vi "Calculate Average Center.vi"(10 "Position":i32, 11 "Gantry Fiducials":dbl[](array[numeric])) -> (2 "Array":cluster{"X":sgl, "Y":sgl}[](array[cluster]), 3 "XYZTheta":dbl[](array[numeric]))   [LabVIEW 2020, in "Assembly Tray.lvclass"]
uses:
  Assembly Tray.lvclass
  <vilib>/Analysis/NI_AALBase.lvlib
  <vilib>/Analysis/baseanly.llb/Mean (DBL).vi
  <vilib>/vision/NI_Vision_Development_Module.lvlib
panel:
  in  "Line 1":T1
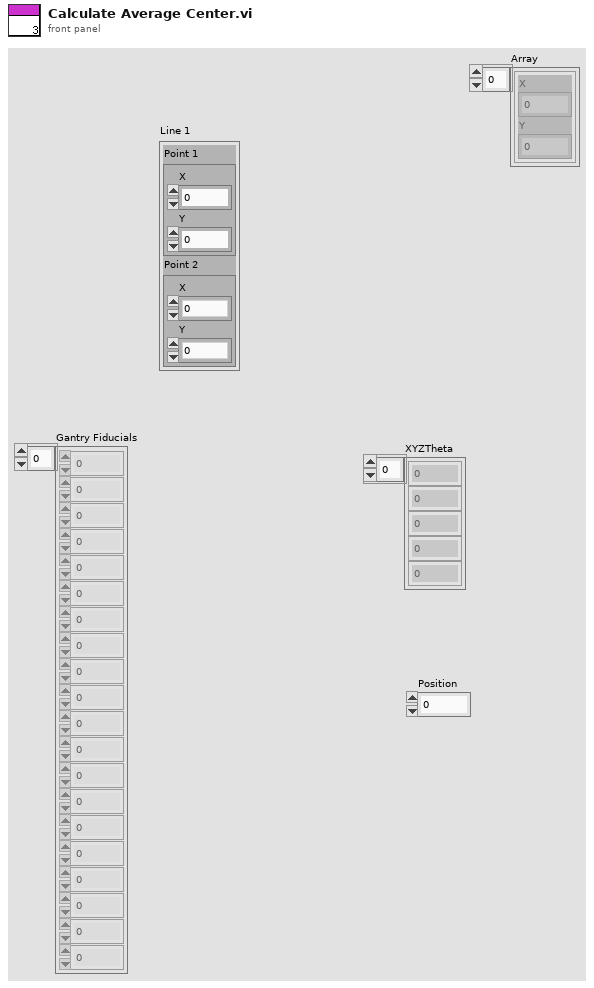
[diagram p1: front panel]
types:
  T1 = cluster{"Point 1":cluster{"X":dbl, "Y":dbl}, "Point 2":cluster{"X":dbl, "Y":dbl}}
  T2 = cluster{"Point 1":cluster{"X":dbl, "Y":dbl}, "Point 2":cluster{"X":dbl, "Y":dbl}}[]
  T3 = cluster{"Point 1":cluster{"X":dbl, "Y":dbl}, "Point 2":cluster{"X":dbl, "Y":dbl}}[][]
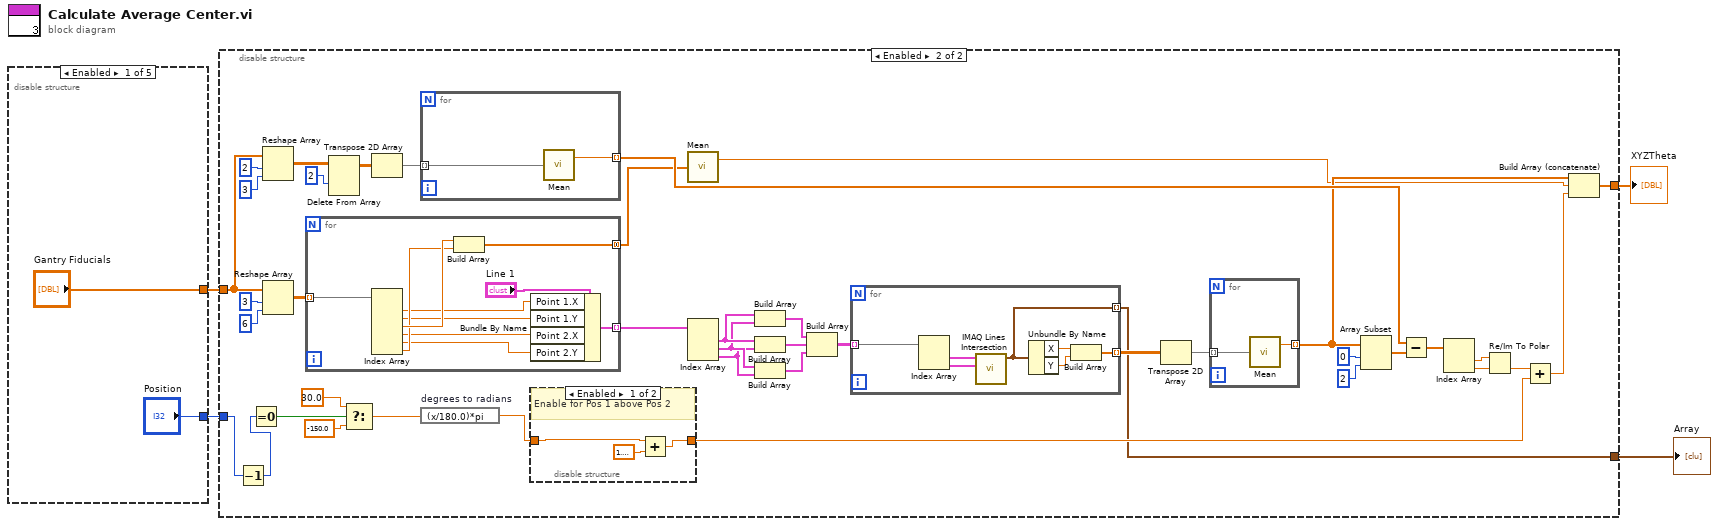
[diagram p0: block diagram]
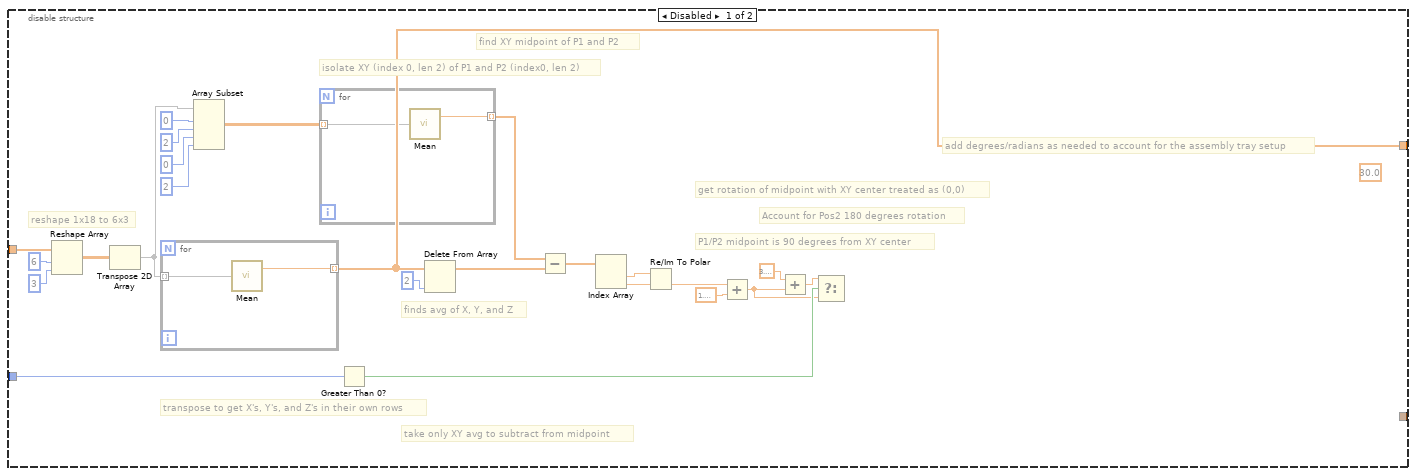
[diagram p2: hidden frame]
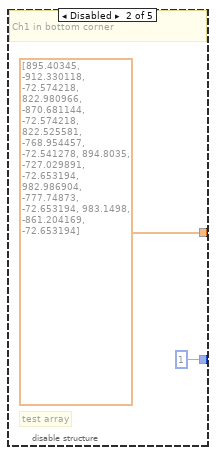
[diagram p4: hidden frame]
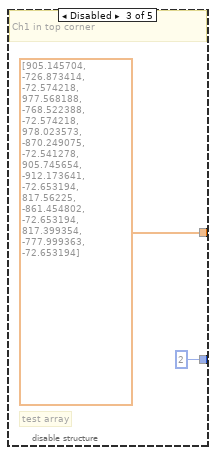
[diagram p5: hidden frame]
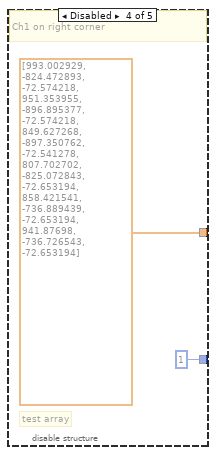
[diagram p6: hidden frame]
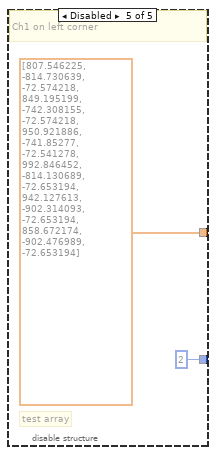
[diagram p7: hidden frame]
diagram:
  n1 = disable-structure shown="Enabled" {
    disable-tunnel: ["Gantry Fiducials" dbl[] [895.40345, -912.330118, -72.574218, 822.980966, -870.681144, -72.574218, 822.525581, -768.954457, -72.541278, 894.8035, -727.029891, -72.653194, 982.986904, -777.74873, -72.653194, 983.1498, -861.204169, -72.653194] dbl[] [905.145704, -726.873414, -72.574218, 977.568188, -768.522388, -72.574218, 978.023573, -870.249075, -72.541278, 905.745654, -912.173641, -72.653194, 817.56225, -861.454802, -72.653194, 817.399354, -777.999363, -72.653194] dbl[] [993.002929, -824.472893, -72.574218, 951.353955, -896.895377, -72.574218, 849.627268, -897.350762, -72.541278, 807.702702, -825.072843, -72.653194, 858.421541, -736.889439, -72.653194, 941.87698, -736.726543, -72.653194] dbl[] [807.546225, -814.730639, -72.574218, 849.195199, -742.308155, -72.574218, 950.921886, -741.85277, -72.541278, 992.846452, -814.130689, -72.653194, 942.127613, -902.314093, -72.653194, 858.672174, -902.476989, -72.653194]] -> w4
    disable-tunnel: ["Position" 1 ("Position") 2 ("Position") 1 ("Position") 2 ("Position")] -> w2
    frame Enabled {
    }
    frame Disabled {
      # "test array"
      # "Ch1 in bottom corner"
    }
    frame Disabled {
      # "test array"
      # "Ch1 in top corner"
    }
    frame Disabled {
      # "test array"
      # "Ch1 on right corner"
    }
    frame Disabled {
      # "test array"
      # "Ch1 on left corner"
    }
  }
  n2 = disable-structure shown="Enabled" {
    disable-tunnel: [w32 w64] -> w3
    disable-tunnel: w4 -> [w19 w56]
    disable-tunnel: w2 -> [w15 w46]
    disable-tunnel: [_ w44] -> w1
    frame Disabled {
      (unwired) 30.0
      # "reshape 1x18 to 6x3"
      # "transpose to get X's, Y's, and Z's in their own rows"
      # "Account for Pos2 180 degrees rotation"
      # "P1/P2 midpoint is 90 degrees from XY center"
      # "add degrees/radians as needed to account for the assembly tray setup"
      # "get rotation of midpoint with XY center treated as (0,0)"
      # "take only XY avg to subtract from midpoint"
      # "find XY midpoint of P1 and P2"
      # "isolate XY (index 0, len 2) of P1 and P2 (index0, len 2)"
      # "finds avg of X, Y, and Z"
      n3 = Reshape Array(w19, 6 ("dimension size"), 3 ("dimension size")) -> (w16:dbl[][])
      n4 = Transpose 2D Array(2D array=w16) -> (transposed array=w20:dbl[][])
      n5 = for {
        tunnel: [w43] -> w32 mode=indexing
        tunnel: w20 -> [w42] mode=indexing
        n6 = call-poly <vilib>:"Mean.vi"("X"=w42) -> ("mean"=w43:dbl)  [unwired: 1 out]
      }
      n7 = Array Subset(array=w20, index (row)=0 ("index"), length (row)=2 ("length"), index (col)=0 ("index"), length (col)=2 ("length")) -> (w33:dbl[][])
      n8 = for {
        tunnel: [w41] -> w29 mode=indexing
        tunnel: w33 -> [w40] mode=indexing
        n9 = call-poly <vilib>:"Mean.vi"("X"=w40) -> ("mean"=w41:dbl)  [unwired: 1 out]
      }
      n10 = Greater Than 0?(x=w15) -> (x > 0?=w25:bool)
      n11 = Delete From Array(array=w32, index=2) -> (array with subset deleted=w30:dbl[])  [unwired: 1 in, 1 out]
      n12 = Subtract(x=w29, y=w30) -> (x-y=w28:dbl[])
      n13 = Index Array(array=w28) -> (element #1=w39:dbl, element #2=w38:dbl)  [unwired: 2 in]
      n14 = Re/Im To Polar(2:w38, 3:w39) -> (0:w27:dbl)  [unwired: 1 out]
      n15 = Add(x=w27, y=1.5707963267948966) -> (x+y=w22:dbl)
      n16 = Add(x=3.141592653589793, y=w22) -> (x+y=w24:dbl)
      n17 = Select(t=w24, s=w25, f=w22) -> (s? t:f=w21:dbl)
    }
    frame Enabled {
      n18 = Decrement(x=w46) -> (x-1=w47:i32)
      n19 = Equal To 0?(x=w47) -> (x = 0?=w54:bool)
      n20 = Reshape Array(w56, 2 ("dimension size"), 3 ("dimension size")) -> (w60:dbl[][])
      n21 = Reshape Array(w56, 3 ("dimension size"), 6 ("dimension size")) -> (w82:dbl[][])
      n22 = for {
        tunnel: w82 -> [w105] mode=indexing
        tunnel: [w102] -> w66 mode=concatenating
        tunnel: [w97] -> w74 mode=indexing
        n23 = Index Array(array=w105) -> (element #1=w101:dbl, element #2=w100:dbl, element #3=w104:dbl, element #4=w99:dbl, element #5=w98:dbl, element #6=w103:dbl)  [unwired: 6 in]
        n24 = Build Array(w104, w103) -> (w102:dbl[])
        n25 = Bundle By Name(cluster="Line 1", "Point 1.X"=w101, "Point 1.Y"=w100, "Point 2.X"=w99, "Point 2.Y"=w98) -> (w97:T1)
      }
      n26 = Delete From Array(array=w60, index (row)=2) -> (array with subset deleted=w58:dbl[][])  [unwired: 2 in, 1 out]
      n27 = Select(t=30.0, s=w54, f=-150.0) -> (s? t:f=w50:dbl)
      n28 = Transpose 2D Array(2D array=w58) -> (transposed array=w81:dbl[][])
      n29 = for {
        tunnel: w81 -> [w108] mode=indexing
        tunnel: [w107] -> w80 mode=indexing
        n30 = call-poly <vilib>:"Mean.vi"("X"=w108) -> ("mean"=w107:dbl)  [unwired: 1 out]
      }
      n31 = expression code="(x/180.0)*pi" "degrees to radians"(w50) -> (w49:dbl)
      n32 = disable-structure shown="Enabled" {
        disable-tunnel: w49 -> [w87 w89]
        disable-tunnel: [w88 w89] -> w48
        frame Enabled {
          # "Enable for Pos 1 above Pos 2"
          n33 = Add(x=w87, y=1.5707963267948966) -> (x+y=w88:dbl)
        }
        frame Disabled {
          # "Enable for Pos1 left of Pos2"
        }
      }
      n34 = call-poly <vilib>:"Mean.vi"("X"=w66) -> ("mean"=w63:dbl)  [unwired: 1 out]
      n35 = Index Array(array=w74) -> (element #1=w73:T1, element #2=w72:T1, element #3=w71:T1)  [unwired: 3 in]
      n36 = Build Array(w73, w72) -> (w70:T2)
      n37 = Build Array(w73, w71) -> (w69:T2)
      n38 = Build Array(w72, w71) -> (w68:T2)
      n39 = Build Array(w70, w69, w68) -> (w67:T3)
      n40 = for {
        tunnel: w67 -> [w96] mode=indexing
        tunnel: [w91] -> w45 mode=indexing
        tunnel: [w90] -> w44 mode=indexing
        n41 = Index Array(array=w96) -> (element #1=w95:T1, element #2=w94:T1)  [unwired: 2 in]
        n42 = call "IMAQ Lines Intersection"("Line 2"=w94, "Line 1"=w95) -> ("Intersection Point"=w90:cluster{"X":sgl, "Y":sgl})  [unwired: 7 in, 2 out]
        n43 = Unbundle By Name(w90) -> ("X"=w93:sgl, "Y"=w92:sgl)
        n44 = Build Array(w93, w92) -> (w91:sgl[])
      }
      n45 = Transpose 2D Array(2D array=w45) -> (transposed array=w75:sgl[][])
      n46 = for {
        tunnel: w75 -> [w110] mode=indexing
        tunnel: [w109] -> w65 mode=indexing
        n47 = call-poly <vilib>:"Mean.vi"("X"=w110) -> ("mean"=w109:dbl)  [unwired: 1 out]
      }
      n48 = Array Subset(array=w65, index=0, length=2) -> (w57:dbl[])
      n49 = Subtract(x=w80, y=w57) -> (x-y=w83:dbl[])
      n50 = Index Array(array=w83) -> (element #1=w77:dbl, element #2=w76:dbl)  [unwired: 2 in]
      n51 = Re/Im To Polar(2:w76, 3:w77) -> (0:w53:dbl)  [unwired: 1 out]
      n52 = Add(x=w53, y=w48) -> (x+y=w52:dbl)
      n53 = Build Array (concatenate)(w65, w63, w52) -> (w64:dbl[])
    }
  }
  "XYZTheta" <- w3
  "Array" <- w1
